vi "Test TDM writeread file Query with Result.vi"(8 "error in (no error)":errorcluster, 10 "Search Parameters":T2[](array[typedef])=[{"eSearch Types"=enum."eSearchFile", "Property Name"="Test", "DataFinder Comparisons"=enum."=", "Property Value"="test"}], 11 "eSearch Type":T1) -> (0 "error out":errorcluster, 1 "Result TDM":path, 2 "Number of Items":i32, 3 "Results":string[][](array[string]), 4 "Data Returned?":bool)   [LabVIEW 2011]
uses:
  eSearch Types.ctl
  DataFinder Comparisons.ctl
  Datafinder Query.ctl
panel:
  in  "Case Constant\n(See Context Help)":bool=TRUE
  in  "Path":path=path "I:/Engineering/Development/SPARTAN/DATA/TDM"
  in  "Iterations":i32=20
  out "iteration":i32
  # "The query passes back an array of [ Filepath, MN, SN, RunID, CHID, Cond1, ... CondN] per row."
  # "I:\\Engineering\\Development\\SPARTAN\\DATA\\TDM\\Prompted Inputs_4_MI123.tdm"
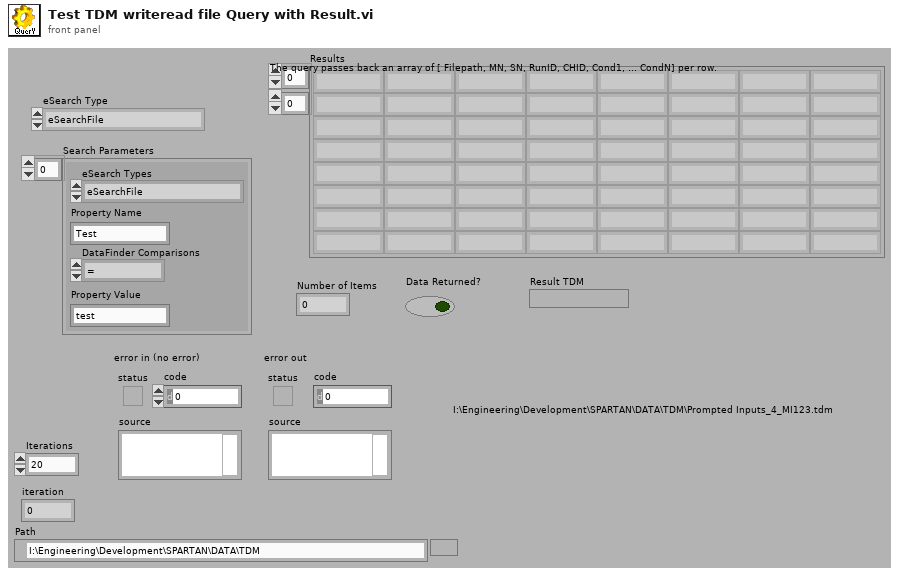
[diagram p1: front panel]
types:
  T1 = typedef "eSearch Types.ctl" = enum16{"eSearchFile", "eSearchChannelGroup", "eSearchChannel"}
  T2 = typedef "Datafinder Query.ctl" = cluster{"eSearch Types":T1, "Property Name":string, "DataFinder Comparisons":T3, "Property Value":string}
  T3 = typedef "DataFinder Comparisons.ctl" = enum16{"=", "<>", "<", "<=", ">", ">="}
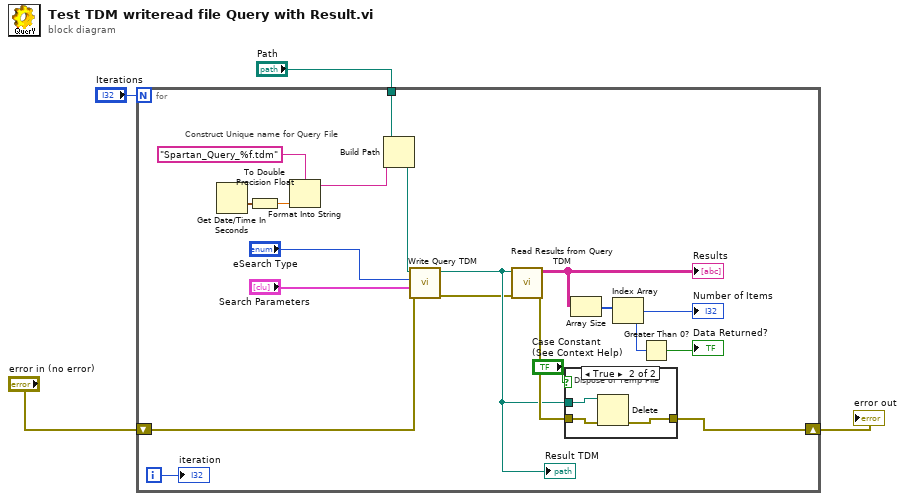
[diagram p0: block diagram]
diagram:
  n1 = for {
    N: "Iterations" -> [_]
    tunnel: "Path" -> [w11]
    shift-right: [w6] -> w3
    shift-left: "error in (no error)" -> [w7]
    i -> [w5]
    # "Construct Unique name for Query File"
    n2 = Get Date/Time In Seconds() -> (seconds since 1Jan1904=w18:timestamp)
    n3 = To Double Precision Float(number=w18) -> (double precision float=w17:dbl)
    n4 = Format Into String(format string="Spartan_Query_%f.tdm", w17) -> (resulting string=w12:string)  [unwired: 2 in, 1 out]
    n5 = Build Path(base path=w11, name or relative path=w12) -> (appended path=w10:path)
    n6 = call "Write Query TDM.vi"("error in (no error)"=w7, "DataFinder parameters"="Search Parameters", "Return Type (ChannelGroup)"="eSearch Type", "Query Path"=w10) -> ("error out"=w8:errorcluster, "Query Path Out"=w9:path)  [unwired: 6 in]
    "Result TDM" <- w9
    n7 = call "Read Results from Query TDM.vi"("error in (no error)"=w8, "Query Path"=w9) -> ("error out"=w14:errorcluster, "Results"=w21:string[][])  [unwired: 8 in]
    "Results" <- w21
    n8 = case shown="True" "Case Constant\n(See Context Help)" {
      tunnel: w14 -> [w24 w27]
      tunnel: [w24 w26] -> w6
      tunnel: w9 -> [_ w25]
      frame False {
      }
      frame True {
        # "Dispose of Temp File"
        n9 = Delete(path (use dialog)=w25, error in=w27) -> (error out=w26:errorcluster)  [unwired: 3 in, 2 out]
      }
    }
    n10 = Array Size(array=w21) -> (size(s)=w20:i32[])
    n11 = Index Array(array=w20) -> (element=w16:i32)  [unwired: 1 in]
    "Number of Items" <- w16
    n12 = Greater Than 0?(x=w16) -> (x > 0?=→"Data Returned?":bool)
    "iteration" <- w5
  }
  "error out" <- w3
